vi "tcp_server.vi"() -> ()   [LabVIEW 2018]
panel:
  out "Waveform Chart":u32(graph)
  out "x-y":u32
  out "concatenated string":string
  out "error out 3":errorcluster
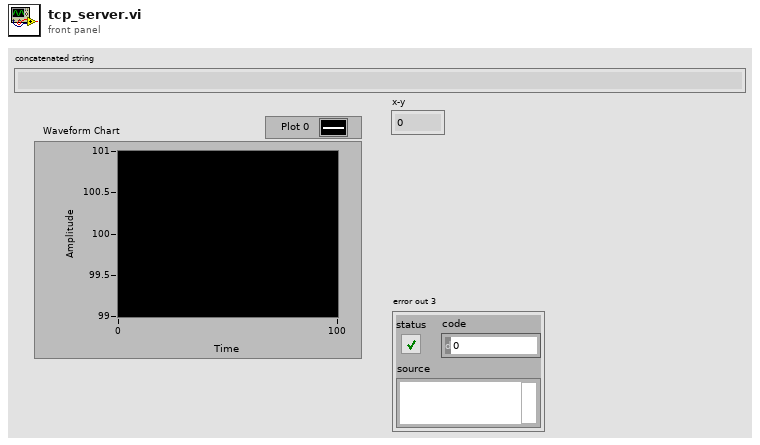
[diagram p1: front panel]
types:
  T1 = enum16{"Standard", "Buffered", "CRLF", "Immediate"}
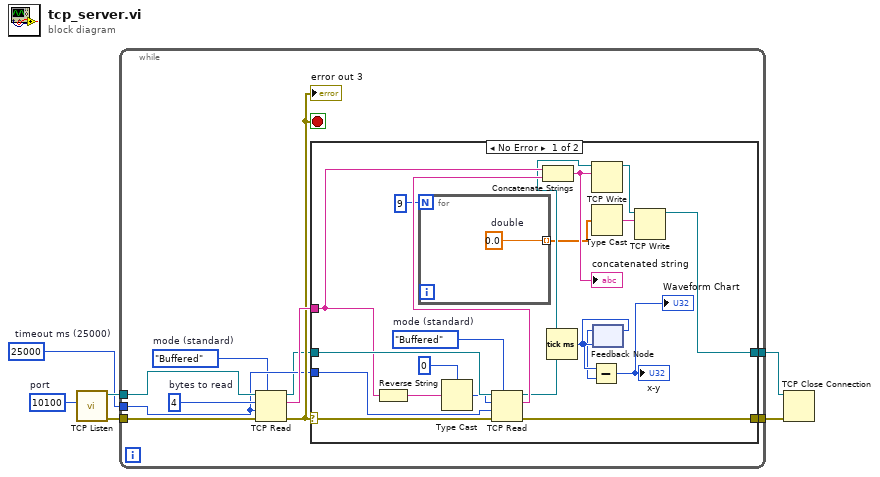
[diagram p0: block diagram]
diagram:
  w2 = 25000  # timeout ms (25000)
  w6 = u16 10100  # port
  n1 = call <vilib>:"TCP Listen.vi"("port"=w6) -> ("error out"=w4:errorcluster, "connection ID"=w5:refnum<k5>)  [unwired: 6 in, 3 out]
  n2 = while {
    tunnel: w5 -> [w16]
    tunnel: w4 -> [w15]
    tunnel: [w9] -> w3
    tunnel: w2 -> [w11]
    tunnel: [w8] -> w1
    stop <- w12 stop-if-true
    w7 = T1."Buffered"  # mode (standard)
    w14 = 4  # bytes to read
    n3 = TCP Read(connection ID=w16, bytes to read=w14, error in (no error)=w15, 7:w7, 9:w11) -> (connection ID out=w10:refnum<k5>, data out=w13:string, error out=w12:errorcluster)
    "error out 3" <- w12
    n4 = case shown="No Error" w12 {
      selector: w12 -> [w31 w38]
      tunnel: w13 -> [w29 _]
      tunnel: w10 -> [w36 w39]
      tunnel: w11 -> [w33 _]
      tunnel: [w23 w39] -> w9
      tunnel: [w30 w38] -> w8
      frame No Error {
        w27 = T1."Buffered"  # mode (standard)
        n5 = Reverse String(1:w29) -> (0:w35:string)
        n6 = for {
          N: 9 -> [_]
          tunnel: [w37] -> w22 mode=indexing
          w37 = 0.0  # double
        }
        n7 = Type Cast(type=0, x=w35) -> (*(type *) &x=w34:i32)
        n8 = TCP Read(connection ID=w36, bytes to read=w34, error in (no error)=w31, 7:w27, 9:w33) -> (connection ID out=w26:refnum<k5>, data out=w28:string, error out=w30:errorcluster)
        n9 = Concatenate Strings(w29, w28) -> (w25:string)
        "concatenated string" <- w25
        n10 = Tick Count (ms)() -> (millisecond timer value=w19:u32)
        n11 = TCP Write(connection ID=w26, data in=w25) -> (connection ID out=w24:refnum<k5>)  [unwired: 2 in, 2 out]
        n12 = Type Cast(x=w22) -> (*(type *) &x=w20:string)  [unwired: 1 in]
        n13 = feedback #1(w19) -> (w18:u32)
        n14 = Subtract(x=w19, y=w18) -> (x-y=→"x-y" →"Waveform Chart":u32)
        n15 = feedback-in #1(w19) -> ()
        n16 = TCP Write(connection ID=w24, data in=w20) -> (connection ID out=w23:refnum<k5>)  [unwired: 2 in, 2 out]
      }
      frame Error {
      }
    }
  }
  n17 = TCP Close Connection(connection ID=w3, error in (no error)=w1) -> ()  [unwired: 1 in, 2 out]
